vi "testLoopbackGERM.vi"(8 "error in (no error)":errorcluster, 11 "TestCase in":refnum<class "DSF CD GE Reflective Memory System Tests.lvclass">) -> (0 "error out":errorcluster, 3 "TestCase out":refnum<class "DSF CD GE Reflective Memory System Tests.lvclass">)   [LabVIEW 2017, in "DSF CD GE Reflective Memory System Tests.lvclass"]
uses:
  DSF CD GE Reflective Memory System Tests.lvclass
  C:/Program Files (x86)/National Instruments/LabVIEW 2017/vi.lib/addons/_JKI Toolkits/VI Tester/TestCase.llb/TestCase.lvclass
  <vilib>/addons/_JKI Toolkits/VI Tester/TestCase.llb/TestCase.lvclass
  <vilib>/NI VeriStand/Execution/Workspace/NI_VS Workspace ExecutionAPI.lvlib
  b55b5565-dc34-4e51-bcfa-5a6cba25043e.vi
  df0c3853-f0b6-44a9-ad36-32614d313efc.vi
  <vilib>/NI Veristand/Execution/Workspace/NI VeriStand - Set Single Channel Value.vi
  <vilib>/NI Veristand/Execution/Workspace/NI VeriStand - Get Single Channel Value.vi
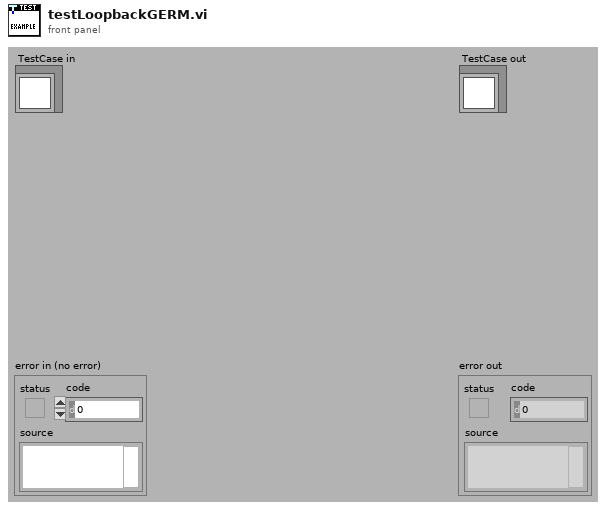
[diagram p1: front panel]
types:
  T1 = typedef "NI_VS Workspace ExecutionAPI.lvlib/WorkspaceAPI.ctl" = refnum<k24>
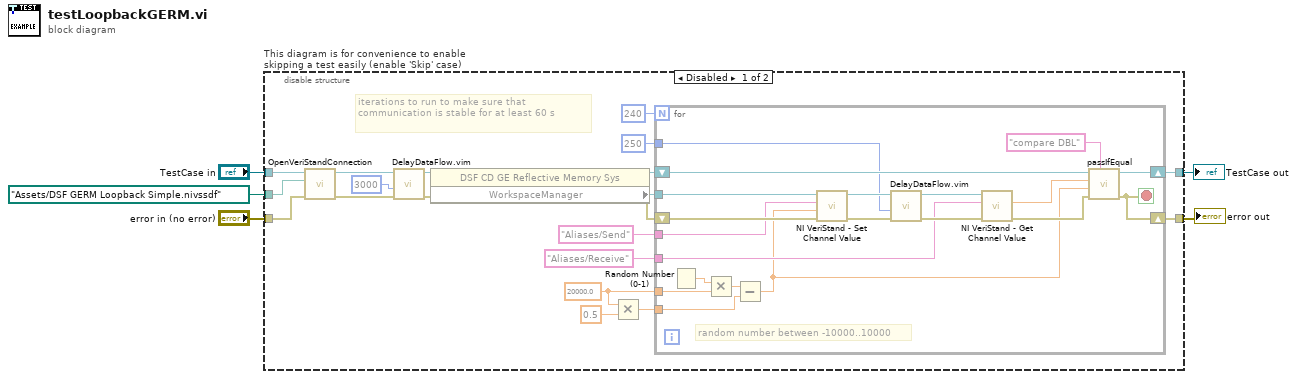
[diagram p0: block diagram]
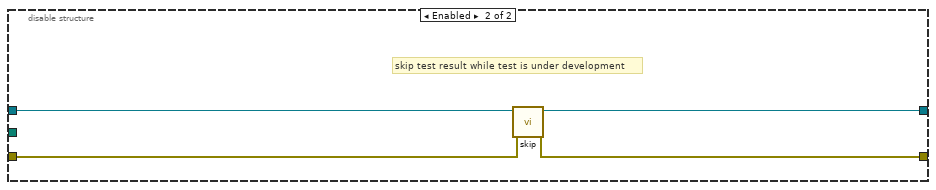
[diagram p2: hidden frame]
diagram:
  n1 = disable-structure "This diagram is for convenience to enable skipping a test easily (enable 'Skip' case)" shown="Disabled" {
    disable-tunnel: "TestCase in" -> [w23 w47]
    disable-tunnel: [w16 w45] -> w2
    disable-tunnel: [w15 w46] -> w4
    disable-tunnel: "error in (no error)" -> [w24 w44]
    disable-tunnel: path "Assets/DSF GERM Loopback Simple.nivssdf" ("System Definition File") -> [w11 _]
    frame Disabled {
      w7 = 20000.0 ("y")
      # "iterations to run to make sure that communication is stable for at least 60 s"
      n2 = call-dynamic "OpenVeriStandConnection.vi"("error in (no error)"=w24, "System Definition File"=w11, "VeriStand Test Case in"=w23) -> ("error out"=w13:errorcluster, "VeriStand Test Case out"=w22:refnum<class "DSF CD GE Reflective Memory System Tests.lvclass">)  [unwired: 6 in, 1 out]
      n3 = call "DelayDataFlow.vim"("value in"=w13, "milliseconds to wait"=u32 3000) -> ("value out"=w12:errorcluster)  [unwired: 2 in, 1 out]
      n4 = property class="DSF CD GE Reflective Memory Sys"(reference=w22, error in=w12) -> (reference out=w17:refnum<class "DSF CD GE Reflective Memory System Tests.lvclass">, error out=w20:errorcluster, "WorkspaceManager"=w21:T1)
      n5 = Multiply(x=w7, y=0.5) -> (x*y=w8:dbl)
      n6 = for {
        N: 240 -> [_]
        tunnel: w21 -> [w43]
        tunnel: "Aliases/Receive" ("Channel") -> [w38]
        tunnel: "Aliases/Send" ("Channel") -> [w37]
        shift-right: [w25] -> w15
        shift-left: w20 -> [w42]
        shift-right: [w33] -> w16
        shift-left: w17 -> [w34]
        tunnel: w8 -> [w28]
        tunnel: w7 -> [w27]
        tunnel: u32 250 ("milliseconds to wait") -> [w26]
        stop <- w25 stop-if-true
        # "random number between -10000..10000"
        n7 = Random Number (0-1)() -> (number: 0 to 1=w32:dbl)
        n8 = Multiply(x=w32, y=w27) -> (x*y=w31:dbl)
        n9 = Subtract(x=w31, y=w28) -> (x-y=w30:dbl)
        n10 = call-poly <vilib>:"NI VeriStand - Set Channel Value.vi"("error in (no error)"=w42, "Value"=w30, "Channel"=w37, "WorkspaceManager in"=w43) -> ("error out"=w41:errorcluster, "WorkspaceManager out"=w39:T1)  [unwired: 6 in]
        n11 = call "DelayDataFlow.vim"("value in"=w41, "milliseconds to wait"=w26) -> ("value out"=w40:errorcluster)  [unwired: 2 in, 1 out]
        n12 = call-poly <vilib>:"NI VeriStand - Get Channel Value.vi"("error in (no error)"=w40, "Channel"=w38, "WorkspaceManager in"=w39) -> ("error out"=w36:errorcluster, "Value"=w35:dbl)  [unwired: 6 in, 1 out]
        n13 = call-dynamic "passIfEqual.vi"("custom report message (\"\")"="compare DBL" ("custom report message (\"\")"), "error in (no error)"=w36, "y"=w30, "x"=w35, "TestCase in"=w34) -> ("error out"=w25:errorcluster, "TestCase out"=w33:refnum<class "DSF CD GE Reflective Memory System Tests.lvclass">)  [unwired: 5 in]
      }
    }
    frame Enabled {
      # "skip test result while test is under development"
      n14 = call <vilib>:"skip.vi"("error in (no error)"=w44, "TestCase in"=w47) -> ("error out"=w46:errorcluster, "TestCase out"=w45:refnum<class "DSF CD GE Reflective Memory System Tests.lvclass">)  [unwired: 8 in]
    }
  }
  "error out" <- w4
  "TestCase out" <- w2
